vi "autonomousDriveFoward.vi"(0 "Four Encoder Values":string[](array[string]), 5 "Deceleration Zone":dbl, 7 "Target Speed":dbl, 9 "Target Distance":dbl, 11 "Constants":dbl[](array[numeric])) -> ()   [LabVIEW 2014]
panel:
  # "Error Proportion"
  # "Left Rear"
  # "Integration of Errors"
  # "Left Front"
  # "Derivative of the Rate"
  # "Right Rear"
  # "Right Front"
  # "Feet Foward"
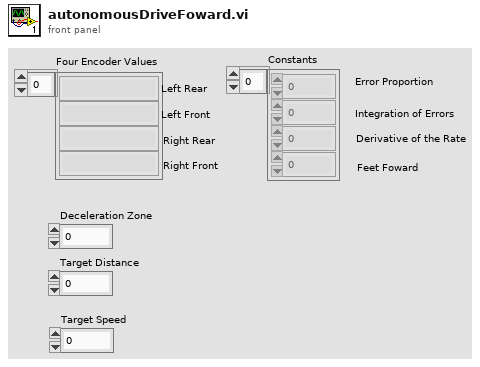
[diagram p1: front panel]
types:
  T1 = typedef "WPI_EncoderDevRef.ctl" = cluster{"DevStatus":errorcluster, "EncoderIndex":T2, "CounterIndex":T3, "DistancePerCount":dbl, "Decoding Type":T4}
  T2 = typedef "FPGA_EncoderIdx.ctl" = enum8{"Enc 0", "Enc 1", "Enc 2", "Enc 3", "Enc 4", "Enc 5", "Enc 6", "Enc 7", "Invalid"}
  T3 = typedef "FPGA_CounterCtrSystemIndex.ctl" = enum8{"Ctr 0", "Ctr 1", "Ctr 2", "Ctr 3", "Ctr 4", "Ctr 5", "Ctr 6", "Ctr 7", "Invalid"}
  T4 = typedef "WPI_EncoderType.ctl" = enum16{"1x", "2x", "4x"}
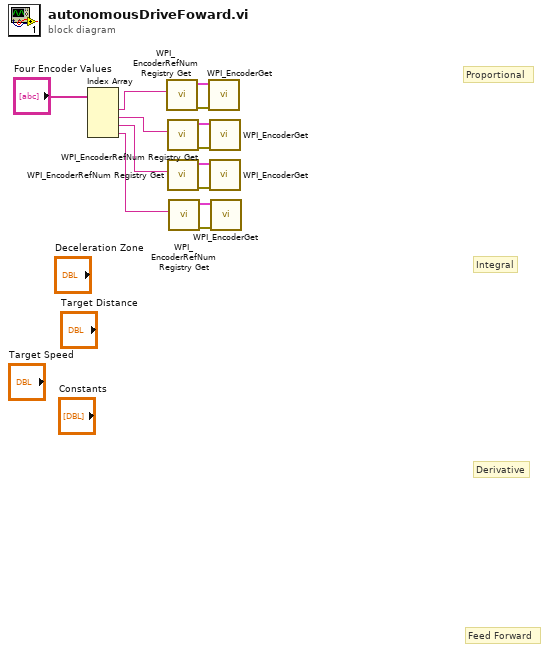
[diagram p0: block diagram]
diagram:
  # "Feed Forward"
  # "Derivative"
  # "Integral"
  # "Proportional"
  n1 = Index Array(array="Four Encoder Values") -> (element #1=w7:string, element #2=w6:string, element #3=w5:string, element #4=w4:string)  [unwired: 4 in]
  n2 = call <vilib>:"WPI_EncoderRefNum Registry Get.vi"("refnum name"=w7) -> ("error out"=w12:errorcluster, "EncoderDevRef"=w11:T1)  [unwired: 9 in]
  n3 = call <vilib>:"WPI_EncoderRefNum Registry Get.vi"("refnum name"=w6) -> ("error out"=w10:errorcluster, "EncoderDevRef"=w3:T1)  [unwired: 9 in]
  n4 = call <vilib>:"WPI_EncoderRefNum Registry Get.vi"("refnum name"=w5) -> ("error out"=w9:errorcluster, "EncoderDevRef"=w2:T1)  [unwired: 9 in]
  n5 = call <vilib>:"WPI_EncoderRefNum Registry Get.vi"("refnum name"=w4) -> ("error out"=w8:errorcluster, "EncoderDevRef"=w1:T1)  [unwired: 9 in]
  n6 = call <vilib>:"WPI_EncoderGet.vi"("error in (no error)"=w12, "EncoderDevRef"=w11) -> ()  [unwired: 4 in, 6 out]
  n7 = call <vilib>:"WPI_EncoderGet.vi"("error in (no error)"=w10, "EncoderDevRef"=w3) -> ()  [unwired: 4 in, 6 out]
  n8 = call <vilib>:"WPI_EncoderGet.vi"("error in (no error)"=w9, "EncoderDevRef"=w2) -> ()  [unwired: 4 in, 6 out]
  n9 = call <vilib>:"WPI_EncoderGet.vi"("error in (no error)"=w8, "EncoderDevRef"=w1) -> ()  [unwired: 4 in, 6 out]
